vi "Tic Toc.vi"(8 "error in (no error)":errorcluster, 11 "Last Tic":u32) -> (0 "error out":errorcluster, 2 "Consumed ticks":u32, 3 "New Toc":u32)   [LabVIEW 2016]
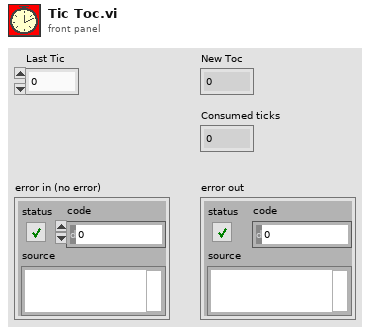
[diagram p1: front panel]
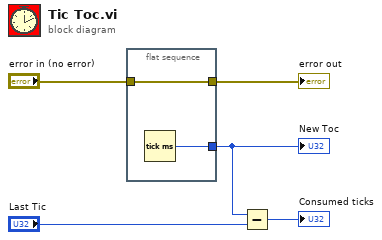
[diagram p0: block diagram]
diagram:
  n1 = flat-sequence {
    tunnel: [w7] -> w2
    tunnel: "error in (no error)" -> [w6]
    tunnel: [w6] -> w4
    frame #0 {
      n2 = Tick Count (ms)() -> (millisecond timer value=w7:u32)
    }
  }
  n3 = Subtract(x=w2, y="Last Tic") -> (x-y=→"Consumed ticks":u32)
  "New Toc" <- w2
  "error out" <- w4
